vi "Write current execution time.vi"(8 "error in (no error)":errorcluster, 10 "current execution time (us)":u32, 11 "Execution Unit in":refnum<class "Execution Unit.lvclass">) -> (0 "error out":errorcluster, 3 "Execution Unit out":refnum<class "Execution Unit.lvclass">)   [LabVIEW 2020, in "Ballard MIL-STD-1553 Engine.lvlib" / "Implementation.lvlib" / "Execution Unit.lvclass"]
uses:
  Execution Unit.lvclass
  Execution Unit.lvclass/Execution Unit.ctl
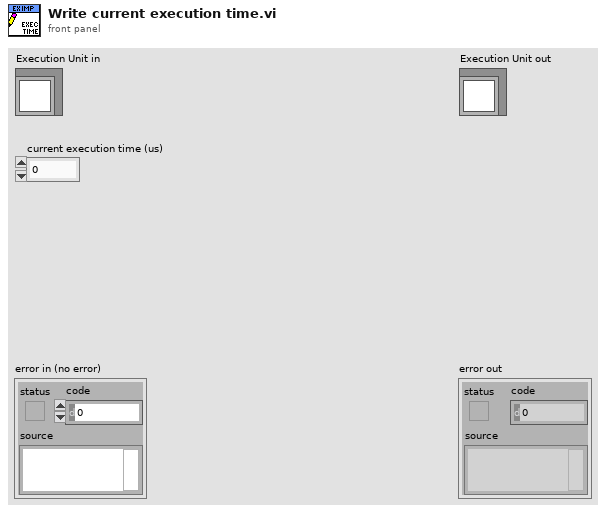
[diagram p1: front panel]
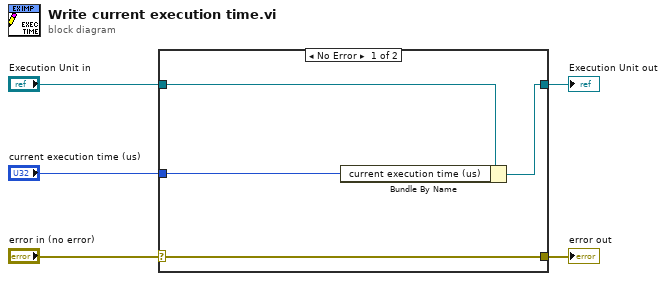
[diagram p0: block diagram]
diagram:
  n1 = case shown="No Error" "error in (no error)" {
    selector: "error in (no error)" -> [w9 w10]
    tunnel: [w9 w10] -> w4
    tunnel: [w7 w11] -> w2
    tunnel: "Execution Unit in" -> [w8 w11]
    tunnel: "current execution time (us)" -> [w6 _]
    frame No Error {
      n2 = Bundle By Name(cluster=w8, "current execution time (us)"=w6) -> (w7:refnum<class "Execution Unit.lvclass">)
    }
    frame Error {
    }
  }
  "error out" <- w4
  "Execution Unit out" <- w2
